vi "UI Main.vi"() -> ()   [LabVIEW 2013]
uses:
  controls/Control Configuration.ctl
  controls/UI Data.ctl
  controls/All FPGA Configuration Values.ctl
  controls/FPGA State.ctl
  controls/Raw Values.ctl
  Globals/Global - All UI Loop Stop.vi
  Globals/Global - UI Stream and Variable Connections.vi
  Globals/Global - Configuration Options.vi
  support/User Event - Stop/User Event - Stop.lvlib
  support/Message Queue/Message Queue.lvlib
panel:
  out "crio-9075-01.me.wisc.edu":string="128.104.188.88"
  in  "Switch to Safe State":bool
  in  "Exit":bool
  out "System Status":string
  out "Current FPGA Control Mode":u16(ring) items=["Safe State", "Manual", "Control (PID)"]
  in  "Settings Tab":T1(tab)
  in  "Channel 3 Setpoint":fxp<+/-,16,5>
  in  "Channel 2 Setpoint":fxp<+/-,16,5>
  in  "Channel 1 Setpoint":fxp<+/-,16,5>
  in  "Channel 0 Setpoint":fxp<+/-,16,5>
  in  "Update Control Configuration":bool
  in  "Control Configurations":T2[](array[typedef])
  in  "Run Control":bool
  in  "Stop Control":bool
  in  "Custom Controller Inputs":T3
  in  "Channel 3 Manual Value":fxp<+/-,16,5>
  in  "Channel 2 Manual Value":fxp<+/-,16,5>
  in  "Channel 1 Manual Value":fxp<+/-,16,5>
  in  "Channel 0 Manual Value":fxp<+/-,16,5>
  in  "Run Manual":bool
  in  "Stop Manual":bool
  out "Input Values":T4(graph)
  out "Output Values":T4(graph)
  out "Actual Loop Period (ticks)":u32
  out "Largest Contiguous Memory (bytes)":dbl(graph)
  out "CPU Usage (%)":dbl(graph)
  out "Connected?":bool
  in  "Connect to Controller":bool
  in  "Controller Address":string="128.104.188.88"
  # "LabVIEW FPGA Control on CompactRIO"
  # "Position Command"
  # "Connection Settings"
  # "Force Command"
  # "Element 0 - Chan 0\nElement 1 - Chan 1\nElement 2 - Chan 2\nElement 3 - Chan 3"
  # "Setpoint changes are sent to the target automatically."
  # "Control Configuration changes are sent to the target when you click \"Update Control Configurations\"."
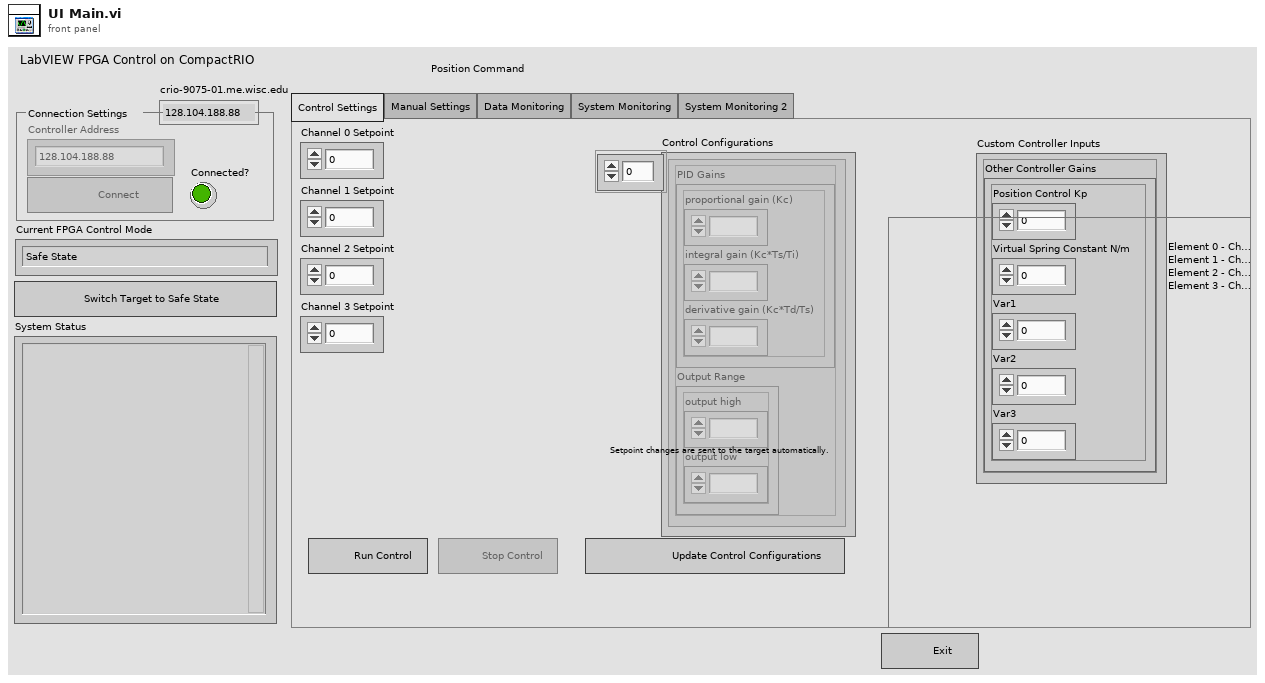
[diagram p1: front panel]
types:
  T1 = enum32{"Control Settings", "Manual Settings", "Data Monitoring", "System Monitoring", "System Monitoring 2"}
  T2 = typedef "Control Configuration.ctl" = cluster{"PID Gains":cluster{"proportional gain (Kc)":fxp<+/-,16,8>, "integral gain (Kc*Ts/Ti)":fxp<+/-,16,8>, "derivative gain (Kc*Td/Ts)":fxp<+/-,16,8>}, "Output Range":cluster{"output high":fxp<+/-,16,5>, "output low":fxp<+/-,16,5>}}
  T3 = cluster{"Other Controller Gains":cluster{"Position Control Kp":fxp<+/-,16,8>, "Virtual Spring Constant N/m":fxp<+/-,16,8>, "Var1":fxp<+/-,16,8>, "Var2":fxp<+/-,16,5>, "Var3":fxp<+/-,16,5>}}
  T4 = cluster{"Channel 0":dbl, "Channel 1":dbl, "Channel 2":dbl, "Channel 3":dbl}
  T5 = typedef "UI Data.ctl" = cluster{"Switch to Safe State Ref":refnum<vi>, "Run Manual Ref":refnum<vi>, "Stop Manual Ref":refnum<vi>, "Run Control Ref":refnum<vi>, "Stop Control Ref":refnum<vi>, "Update Control Configurations Ref":refnum<vi>, "Ch 0 Setpoint Ref":refnum<vi>, "Ch 1 Setpoint Ref":refnum<vi>, "Ch 2 Setpoint Ref":refnum<vi>, "Ch 3 Setpoint Ref":refnum<vi>, "Ch 0 Manual Ref":refnum<vi>, "Ch 1 Manual Ref":refnum<vi>, "Ch 2 Manual Ref":refnum<vi>, "Ch 3 Manual Ref":refnum<vi>, "Control Configurations Ref":refnum<vi>, "Custom Controller Cluster Ref":refnum<vi>}
  T6 = typedef "Message Queue.lvlib/All Message Queues.ctl" = cluster{"UI":refnum<queue>}
  T7 = cluster{"Channel 0 Setpoint":fxp<+/-,16,5>, "Channel 1 Setpoint":fxp<+/-,16,5>, "Channel 2 Setpoint":fxp<+/-,16,5>, "Channel 3 Setpoint":fxp<+/-,16,5>}
  T8 = cluster{"Channel 0 Manual Value":fxp<+/-,16,5>, "Channel 1 Manual Value":fxp<+/-,16,5>, "Channel 2 Manual Value":fxp<+/-,16,5>, "Channel 3 Manual Value":fxp<+/-,16,5>}
  T9 = cluster{"Message":string, "Message Data":variant}
  T10 = typedef "All FPGA Configuration Values.ctl" = cluster{"FPGA State":T11, "Manual Values":T12, "Setpoints":T12, "Control Configurations":T2[]}
  T11 = typedef "FPGA State.ctl" = enum16{"Safe State", "Manual", "Control (PID)"}
  T12 = typedef "Raw Values.ctl" = cluster{"Channel 0":fxp<+/-,20,5>, "Channel 1":fxp<+/-,20,5>, "Channel 2":fxp<+/-,20,5>, "Channel 3":fxp<+/-,20,5>}
  T13 = typedef "Variable References.ctl" = cluster{"CPU Usage":refnum<k21>, "Contiguous Memory":refnum<k21>, "Input Values":refnum<k21>, "Output Values":refnum<k21>, "FPGA Mode":refnum<k21>, "Actual Loop Period":refnum<k21>}
  T14 = cluster{string, "Custom Controller Inputs":cluster{"Other Controller Gains":cluster{"Position Control Kp":fxp<+/-,16,8>, "Virtual Spring Constant N/m":fxp<+/-,16,8>, "Var1":fxp<+/-,16,8>, "Var2":fxp<+/-,16,5>, "Var3":fxp<+/-,16,5>}}}
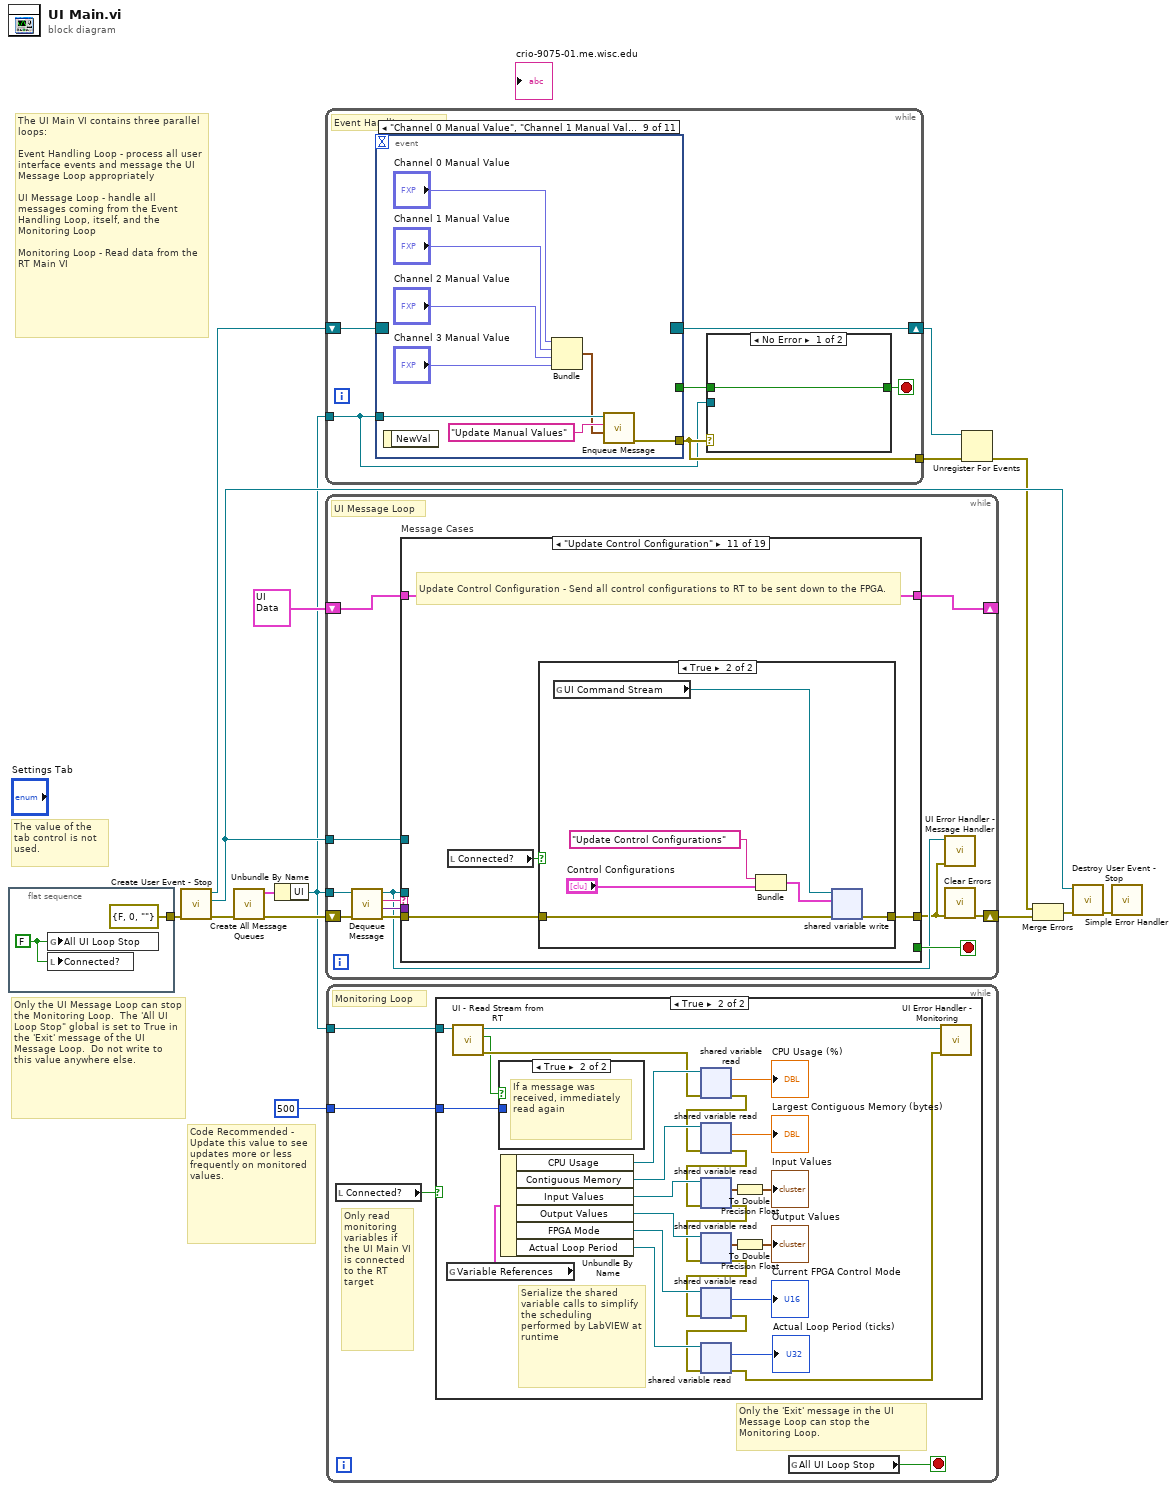
[diagram p0: block diagram]
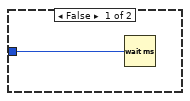
[diagram p2: hidden frame]
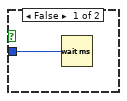
[diagram p3: hidden frame]
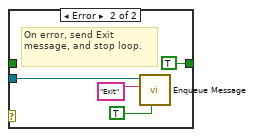
[diagram p4: hidden frame]
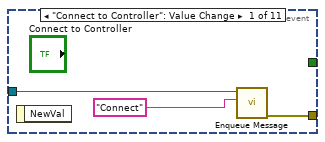
[diagram p5: hidden frame]
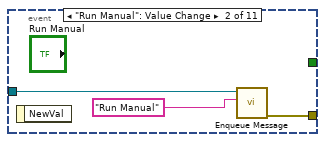
[diagram p6: hidden frame]
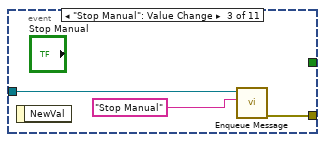
[diagram p7: hidden frame]
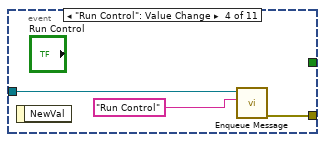
[diagram p8: hidden frame]
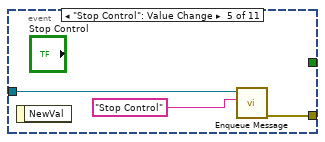
[diagram p9: hidden frame]
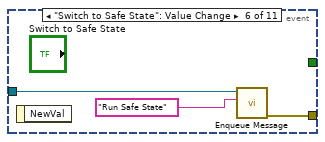
[diagram p10: hidden frame]
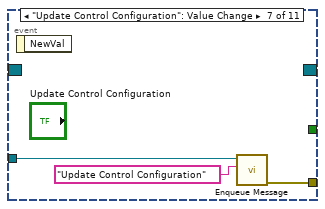
[diagram p11: hidden frame]
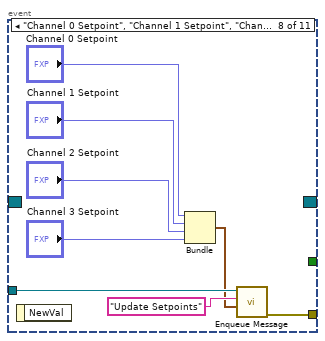
[diagram p12: hidden frame]
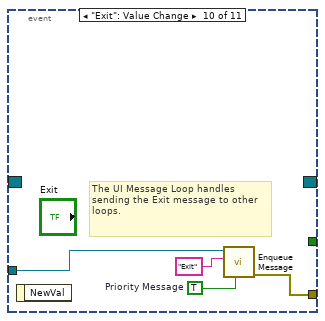
[diagram p13: hidden frame]
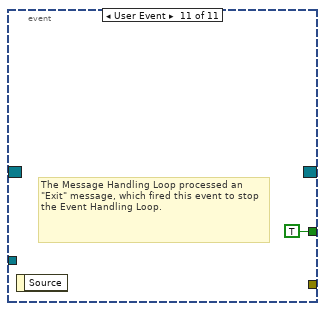
[diagram p14: hidden frame]
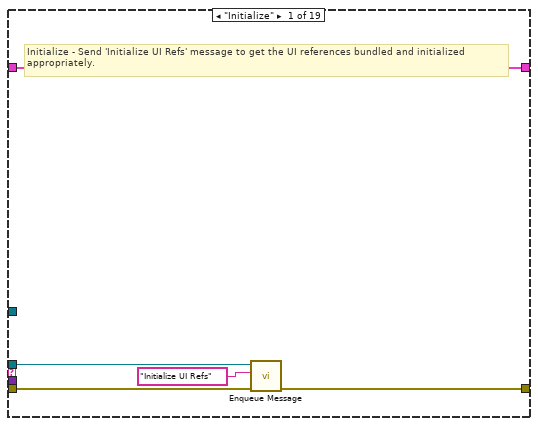
[diagram p15: hidden frame]
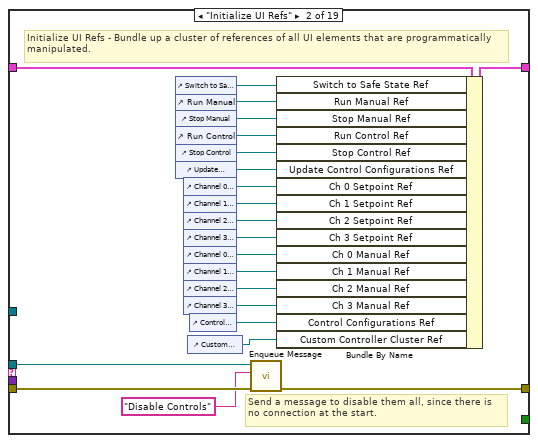
[diagram p16: hidden frame]
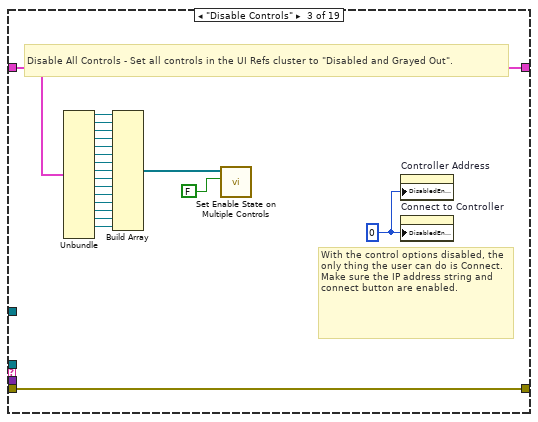
[diagram p17: hidden frame]
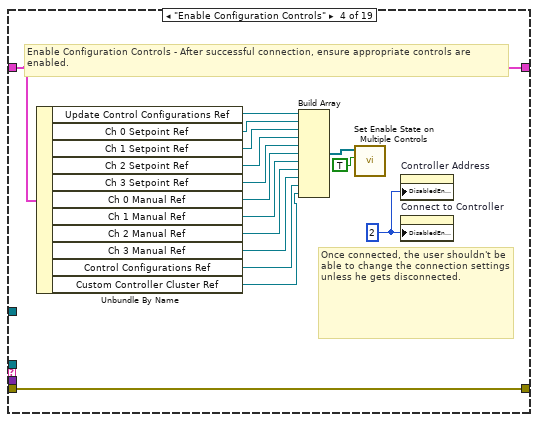
[diagram p18: hidden frame]
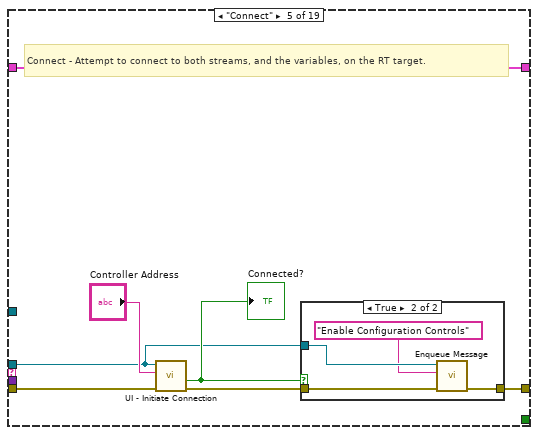
[diagram p19: hidden frame]
diagram:
  # "Code Recommended - Update this value to see updates more or less frequently on monitored values."
  # "The UI Main VI contains three parallel loops:\n\nEvent Handling Loop - process all user interface events and message the UI Message Loop appropriately\n\nUI Message Loop - handle all messages coming from the Event Handling Loop, itself, and the Monitoring Loop\n\nMonitoring Loop - Read data from the RT Main VI"
  # "The value of the tab control is not used."
  # "Only the UI Message Loop can stop the Monitoring Loop.  The 'All UI Loop Stop\" global is set to True in the 'Exit' message of the UI Message Loop.  Do not write to this value anywhere else."
  n1 = flat-sequence {
    tunnel: [errorcluster {"status"=FALSE, "code"=0, "source"=""} ("error in (no error)")] -> w2
    frame #0 {
      w16 = FALSE
      n2 = global write "Global - All UI Loop Stop.vi" "All UI Loop Stop"(w16) -> ()
      n3 = local write "Connected?"(w16) -> ()
    }
  }
  n4 = call "Create User Event - Stop.vi"("error in (no error)"=w2) -> ("error out"=w10:errorcluster, "User Event - Stop"=w11:refnum<user-event>, "Stop Event Registration Refnum"=w12:refnum<event-registration>)  [unwired: 8 in]
  n5 = call "Create All Message Queues.vi"("error in (no error)"=w10) -> ("error out"=w8:errorcluster, "Message Queues out"=w9:T6)  [unwired: 9 in]
  n6 = Unbundle By Name(w9) -> ("UI"=w3:refnum<queue>)
  n7 = while {
    tunnel: w3 -> [w19]
    tunnel: [w21] -> w14
    shift-right: [w18] -> w6
    shift-left: w12 -> [w20]
    stop <- w22 stop-if-true
    # "Event Handling Loop"
    n8 = event shown="[8] \"Channel 0 Manual Value\", \"Channel 1 Manual Value\", \"Channel 2 Manual Value\", \"Channel 3 Manual Value\": Value Change" {
      selector: w20 -> [_ _ _ _ _ _ _ _ _ _ _]
      dyn-events: [_ _ _ _ _ _ _ _ _ _ _] -> w18
      timeout: _ -> [_ _ _ _ _ _ _ _ _ _ _]
      tunnel: [_ _ _ _ _ _ _ _ _ _ TRUE ("Discard?")] -> w23
      tunnel: w19 -> [w29 w32 w35 w38 w41 w44 w49 w52 w61 w66 _]
      tunnel: [w31 w34 w37 w40 w43 w46 w48 w51 w60 w69 _] -> w21
      event "Connect to Controller": Value Change {
        n9 = event-data() -> ()  [unwired: 1 in, 1 out]
        n10 = call "Enqueue Message.vi"("Message"="Connect", "Message Queue"=w29) -> ("error out"=w31:errorcluster)  [unwired: 8 in, 1 out]
      }
      event "Run Manual": Value Change {
        n11 = event-data() -> ()  [unwired: 1 in, 1 out]
        n12 = call "Enqueue Message.vi"("Message"="Run Manual", "Message Queue"=w32) -> ("error out"=w34:errorcluster)  [unwired: 8 in, 1 out]
      }
      event "Stop Manual": Value Change {
        n13 = event-data() -> ()  [unwired: 1 in, 1 out]
        n14 = call "Enqueue Message.vi"("Message"="Stop Manual", "Message Queue"=w35) -> ("error out"=w37:errorcluster)  [unwired: 8 in, 1 out]
      }
      event "Run Control": Value Change {
        n15 = event-data() -> ()  [unwired: 1 in, 1 out]
        n16 = call "Enqueue Message.vi"("Message"="Run Control", "Message Queue"=w38) -> ("error out"=w40:errorcluster)  [unwired: 8 in, 1 out]
      }
      event "Stop Control": Value Change {
        n17 = event-data() -> ()  [unwired: 1 in, 1 out]
        n18 = call "Enqueue Message.vi"("Message"="Stop Control", "Message Queue"=w41) -> ("error out"=w43:errorcluster)  [unwired: 8 in, 1 out]
      }
      event "Switch to Safe State": Value Change {
        n19 = event-data() -> ()  [unwired: 1 in, 1 out]
        n20 = call "Enqueue Message.vi"("Message"="Run Safe State", "Message Queue"=w44) -> ("error out"=w46:errorcluster)  [unwired: 8 in, 1 out]
      }
      event "Update Control Configuration": Value Change {
        n21 = event-data() -> ()  [unwired: 1 in, 1 out]
        n22 = call "Enqueue Message.vi"("Message"="Update Control Configuration", "Message Queue"=w49) -> ("error out"=w48:errorcluster)  [unwired: 8 in, 1 out]
      }
      event "Channel 0 Setpoint", "Channel 1 Setpoint", "Channel 2 Setpoint", "Channel 3 Setpoint": Value Change {
        n23 = event-data() -> ()  [unwired: 1 in, 1 out]
        n24 = Bundle("Channel 0 Setpoint"="Channel 0 Setpoint", "Channel 1 Setpoint"="Channel 1 Setpoint", "Channel 2 Setpoint"="Channel 2 Setpoint", "Channel 3 Setpoint"="Channel 3 Setpoint") -> (w50:T7)  [unwired: 1 in]
        n25 = call "Enqueue Message.vi"("Message Data"=w50, "Message"="Update Setpoints", "Message Queue"=w52) -> ("error out"=w51:errorcluster)  [unwired: 7 in, 1 out]
      }
      event "Channel 0 Manual Value", "Channel 1 Manual Value", "Channel 2 Manual Value", "Channel 3 Manual Value": Value Change {
        n26 = event-data() -> ()  [unwired: 1 in, 1 out]
        n27 = Bundle("Channel 0 Manual Value"="Channel 0 Manual Value", "Channel 1 Manual Value"="Channel 1 Manual Value", "Channel 2 Manual Value"="Channel 2 Manual Value", "Channel 3 Manual Value"="Channel 3 Manual Value") -> (w58:T8)  [unwired: 1 in]
        n28 = call "Enqueue Message.vi"("Message Data"=w58, "Message"="Update Manual Values", "Message Queue"=w61) -> ("error out"=w60:errorcluster)  [unwired: 7 in, 1 out]
      }
      event "Exit": Value Change {
        w67 = TRUE  # Priority Message
        # "The UI Message Loop handles sending the Exit message to other loops."
        n29 = event-data() -> ()  [unwired: 1 in, 1 out]
        n30 = call "Enqueue Message.vi"("Priority Message? (F)"=w67, "Message"="Exit", "Message Queue"=w66) -> ("error out"=w69:errorcluster)  [unwired: 7 in, 1 out]
      }
      event User Event {
        # "The Message Handling Loop processed an \"Exit\" message, which fired this event to stop the Event Handling Loop."
        n31 = event-data() -> ()  [unwired: 1 in, 1 out]
      }
    }
    n32 = case shown="No Error" w21 {
      tunnel: [w24 TRUE ("Discard?")] -> w22
      tunnel: w23 -> [w24 _]
      tunnel: w19 -> [_ w25]
      frame No Error {
      }
      frame Error {
        # "On error, send Exit message, and stop loop."
        n33 = call "Enqueue Message.vi"("Priority Message? (F)"=TRUE ("Discard?"), "Message"="Exit", "Message Queue"=w25) -> ()  [unwired: 7 in, 2 out]
      }
    }
  }
  n34 = while {
    tunnel: w3 -> [w76]
    tunnel: w11 -> [w81]
    shift-right: [w71] -> w15
    shift-left: w8 -> [w80]
    shift-right: [w74] -> _
    shift-left: T5 {"Switch to Safe State Ref"=refnum, "Run Manual Ref"=refnum, "Stop Manual Ref"=refnum, "Run Control Ref"=refnum, "Stop Control Ref"=refnum, "Update Control Configurations Ref"=refnum, "Ch 0 Setpoint Ref"=refnum, "Ch 1 Setpoint Ref"=refnum, "Ch 2 Setpoint Ref"=refnum, "Ch 3 Setpoint Ref"=refnum, "Ch 0 Manual Ref"=refnum, "Ch 1 Manual Ref"=refnum, "Ch 2 Manual Ref"=refnum, "Ch 3 Manual Ref"=refnum, "Control Configurations Ref"=refnum, "Custom Controller Cluster Ref"=refnum} ("Measurement UI Controls") -> [w75]
    stop <- w82 stop-if-true
    # "UI Message Loop"
    n35 = call "Dequeue Message.vi"("error in (no error)"=w80, "Message Queue"=w76) -> ("error out"=w79:errorcluster, "Message Data"=w77:variant, "Message"=w78:string, "dup Message Queue"=w73:refnum<queue>)  [unwired: 6 in]
    n36 = case "Message Cases" shown="\"Update Control Configuration\"" w78 {
      selector: w78 -> [_ _ _ _ _ _ _ _ _ w207 _ _ w250 _ w300 _ _ _ w361]
      tunnel: w73 -> [w84 w91 _ _ w147 _ w165 _ w179 w208 _ _ _ _ w304 _ w346 _ _]
      tunnel: w79 -> [w86 w109 w129 w131 w152 w163 w167 w172 w203 w210 w228 w239 w251 w271 w314 w335 w351 w356 _]
      tunnel: [w85 w92 w129 w131 w146 w163 w166 w171 w182 w209 w227 w238 w252 w270 w315 w333 w352 w355 w359] -> w72
      tunnel: [_ _ _ _ _ _ _ _ _ _ _ _ _ _ _ _ TRUE _ _] -> w82
      tunnel: w77 -> [_ _ _ _ _ _ _ _ w201 _ _ _ w249 w269 w312 w332 _ _ _]
      tunnel: w81 -> [_ _ _ _ _ _ _ _ _ _ _ _ _ _ _ _ w350 _ _]
      tunnel: w75 -> [w87 w108 w128 w142 w151 w162 w169 w173 w198 w211 w229 w240 w253 w268 w316 w334 w348 w354 w357]
      tunnel: [w87 w107 w128 w142 w151 w162 w169 w173 w198 w211 w229 w240 w253 w268 w316 w334 w348 w354 w357] -> w74
      frame "Initialize" {
        # "Initialize - Send 'Initialize UI Refs' message to get the UI references bundled and initialized appropriately."
        n37 = call "Enqueue Message.vi"("error in (no error)"=w86, "Message"="Initialize UI Refs", "Message Queue"=w84) -> ("error out"=w85:errorcluster)  [unwired: 7 in, 1 out]
      }
      frame "Initialize UI Refs" {
        # "Send a message to disable them all, since there is no connection at the start."
        # "Initialize UI Refs - Bundle up a cluster of references of all UI elements that are programmatically manipulated."
        n38 = control-ref of="Switch to Safe State"() -> (w106:refnum<vi>)
        n39 = control-ref of="Run Manual"() -> (w105:refnum<vi>)
        n40 = control-ref of="Stop Manual"() -> (w104:refnum<vi>)
        n41 = control-ref of="Run Control"() -> (w103:refnum<vi>)
        n42 = control-ref of="Stop Control"() -> (w102:refnum<vi>)
        n43 = control-ref of="Update Control Configuration"() -> (w101:refnum<vi>)
        n44 = control-ref of="Channel 0 Setpoint"() -> (w100:refnum<vi>)
        n45 = control-ref of="Channel 1 Setpoint"() -> (w99:refnum<vi>)
        n46 = control-ref of="Channel 2 Setpoint"() -> (w98:refnum<vi>)
        n47 = control-ref of="Channel 3 Setpoint"() -> (w97:refnum<vi>)
        n48 = control-ref of="Channel 0 Manual Value"() -> (w96:refnum<vi>)
        n49 = control-ref of="Channel 1 Manual Value"() -> (w95:refnum<vi>)
        n50 = control-ref of="Channel 2 Manual Value"() -> (w94:refnum<vi>)
        n51 = control-ref of="Channel 3 Manual Value"() -> (w93:refnum<vi>)
        n52 = control-ref of="Custom Controller Inputs"() -> (w88:refnum<vi>)
        n53 = control-ref of="Control Configurations"() -> (w89:refnum<vi>)
        n54 = call "Enqueue Message.vi"("error in (no error)"=w109, "Message"="Disable Controls", "Message Queue"=w91) -> ("error out"=w92:errorcluster)  [unwired: 7 in, 1 out]
        n55 = Bundle By Name(cluster=w108, "Switch to Safe State Ref"=w106, "Run Manual Ref"=w105, "Stop Manual Ref"=w104, "Run Control Ref"=w103, "Stop Control Ref"=w102, "Update Control Configurations Ref"=w101, "Ch 0 Setpoint Ref"=w100, "Ch 1 Setpoint Ref"=w99, "Ch 2 Setpoint Ref"=w98, "Ch 3 Setpoint Ref"=w97, "Ch 0 Manual Ref"=w96, "Ch 1 Manual Ref"=w95, "Ch 2 Manual Ref"=w94, "Ch 3 Manual Ref"=w93, "Control Configurations Ref"=w89, "Custom Controller Cluster Ref"=w88) -> (w107:T5)
      }
      frame "Disable Controls" {
        w110 = 0
        # "With the control options disabled, the only thing the user can do is Connect. Make sure the IP address string and connect button are enabled."
        # "Disable All Controls - Set all controls in the UI Refs cluster to \"Disabled and Grayed Out\"."
        n56 = Unbundle(w128) -> ("Switch to Safe State Ref"=w127:refnum<vi>, "Run Manual Ref"=w126:refnum<vi>, "Stop Manual Ref"=w125:refnum<vi>, "Run Control Ref"=w124:refnum<vi>, "Stop Control Ref"=w123:refnum<vi>, "Update Control Configurations Ref"=w122:refnum<vi>, "Ch 0 Setpoint Ref"=w121:refnum<vi>, "Ch 1 Setpoint Ref"=w120:refnum<vi>, "Ch 2 Setpoint Ref"=w119:refnum<vi>, "Ch 3 Setpoint Ref"=w118:refnum<vi>, "Ch 0 Manual Ref"=w117:refnum<vi>, "Ch 1 Manual Ref"=w116:refnum<vi>, "Ch 2 Manual Ref"=w115:refnum<vi>, "Ch 3 Manual Ref"=w114:refnum<vi>, "Control Configurations Ref"=w113:refnum<vi>)  [unwired: 1 out]
        n57 = Build Array(w127, w126, w125, w124, w123, w122, w121, w120, w119, w118, w117, w116, w115, w114, w113) -> (w112:refnum<vi>[])
        n58 = call "Set Enable State on Multiple Controls.vi"("Enable?"=FALSE, "Controls"=w112) -> ()  [unwired: 10 in]
        n59 = property on="Controller Address" class="Str"("DisabledEnum"=w110) -> ()  [unwired: 2 in, 2 out]
        n60 = property on="Connect to Controller" class="Bool"("DisabledEnum"=w110) -> ()  [unwired: 2 in, 2 out]
      }
      frame "Enable Configuration Controls" {
        w143 = 2
        # "Once connected, the user shouldn't be able to change the connection settings unless he gets disconnected."
        # "Enable Configuration Controls - After successful connection, ensure appropriate controls are enabled."
        n61 = Unbundle By Name(w142) -> ("Update Control Configurations Ref"=w141:refnum<vi>, "Ch 0 Setpoint Ref"=w140:refnum<vi>, "Ch 1 Setpoint Ref"=w139:refnum<vi>, "Ch 2 Setpoint Ref"=w138:refnum<vi>, "Ch 3 Setpoint Ref"=w137:refnum<vi>, "Ch 0 Manual Ref"=w136:refnum<vi>, "Ch 1 Manual Ref"=w135:refnum<vi>, "Ch 2 Manual Ref"=w134:refnum<vi>, "Ch 3 Manual Ref"=w133:refnum<vi>, "Control Configurations Ref"=w132:refnum<vi>, "Custom Controller Cluster Ref"=w130:refnum<vi>)
        n62 = Build Array(w141, w140, w139, w138, w137, w136, w135, w134, w133, w132, w130) -> (w145:refnum<vi>[])
        n63 = call "Set Enable State on Multiple Controls.vi"("Enable?"=TRUE, "Controls"=w145) -> ()  [unwired: 10 in]
        n64 = property on="Controller Address" class="Str"("DisabledEnum"=w143) -> ()  [unwired: 2 in, 2 out]
        n65 = property on="Connect to Controller" class="Bool"("DisabledEnum"=w143) -> ()  [unwired: 2 in, 2 out]
      }
      frame "Connect" {
        # "Connect - Attempt to connect to both streams, and the variables, on the RT target."
        n66 = call "UI - Initiate Connection.vi"("error in (no error)"=w152, "Controller Address"="Controller Address", "Message Queue"=w147) -> ("error out"=w149:errorcluster, "Connected?"=w148:bool)  [unwired: 7 in]
        "Connected?" <- w148
        n67 = case shown="True" w148 {
          tunnel: w149 -> [w153 w157]
          tunnel: w147 -> [_ w156]
          tunnel: [w153 w155] -> w146
          frame False {
          }
          frame True {
            n68 = call "Enqueue Message.vi"("error in (no error)"=w157, "Message"="Enable Configuration Controls", "Message Queue"=w156) -> ("error out"=w155:errorcluster)  [unwired: 7 in, 1 out]
          }
        }
      }
      frame "Close Connections" {
        # "Close Connections - Close the connections shared with the Monitoring Loop."
        n69 = global read "Global - UI Stream and Variable Connections.vi" "UI Command Stream"() -> (w161:refnum<k21>)
        n70 = global read "Global - UI Stream and Variable Connections.vi" "RT Message Stream"() -> (w160:refnum<k21>)
        n71 = global read "Global - UI Stream and Variable Connections.vi" "Variable References"() -> (w159:T13)
        n72 = local write "Connected?"(FALSE ("Connected?")) -> ()
        n73 = Destroy Stream Endpoint(11:w161) -> ()  [unwired: 1 in, 1 out]
        n74 = Destroy Stream Endpoint(11:w160) -> ()  [unwired: 1 in, 1 out]
        n75 = call "Close Variable Connections.vi"("Variable References"=w159) -> ()  [unwired: 11 in]
      }
      frame "Disconnect UI" {
        # "Disconnect UI - Something has gone wrong with the connection. Reinitialize the UI to its disconnected state."
        n76 = local write "Connected?"(FALSE ("Connected?")) -> ()
        n77 = call "Enqueue Message.vi"("error in (no error)"=w167, "Message"="Disable Controls", "Message Queue"=w165) -> ("error out"=w166:errorcluster)  [unwired: 7 in, 1 out]
      }
      frame "Get Settings from FPGA" {
        # "Get Settings from FPGA - Send a command to the RT to retrieve all current FPGA Main VI parameter values and send them back to the UI."
        n78 = local read "Connected?"() -> (w170:bool)
        n79 = case shown="True" w170 {
          tunnel: w172 -> [w174 w178]
          tunnel: [w174 w177] -> w171
          frame False {
            # "Don't bother trying to send a message to the RT system if UI Main VI isn't even connected"
          }
          frame True {
            n80 = global read "Global - UI Stream and Variable Connections.vi" "UI Command Stream"() -> (w175:refnum<k21>)
            n81 = shared-variable-write(w175, w178, T9 {"Message"="Send FPGA Configuration to UI", "Message Data"=variant} ("data in")) -> (w177:errorcluster)  [unwired: 1 in, 2 out]
          }
        }
      }
      frame "Initial UI Values" {
        # "Initial UI Values - These are the current values of the FPGA Main VI's R/W controls. They are used to initialize the panel of UI Main VI upon successful connection to the RT target."
        # "Set values of all manual and setpoint controls via reference."
        n82 = Variant To Data(error in=w203, type=T10 {"FPGA State"=enum."Safe State", "Manual Values"={"Channel 0"=0.0, "Channel 1"=0.0, "Channel 2"=0.0, "Channel 3"=0.0}, "Setpoints"={"Channel 0"=0.0, "Channel 1"=0.0, "Channel 2"=0.0, "Channel 3"=0.0}, "Control Configurations"=[]} ("All FPGA Configuration Values"), Variant=w201) -> (data=w199:T10, error out=w202:errorcluster)
        n83 = Unbundle By Name(w198) -> ("Ch 0 Setpoint Ref"=w193:refnum<vi>, "Ch 1 Setpoint Ref"=w192:refnum<vi>, "Ch 2 Setpoint Ref"=w191:refnum<vi>, "Ch 3 Setpoint Ref"=w190:refnum<vi>, "Ch 0 Manual Ref"=w189:refnum<vi>, "Ch 1 Manual Ref"=w188:refnum<vi>, "Ch 2 Manual Ref"=w187:refnum<vi>, "Ch 3 Manual Ref"=w186:refnum<vi>)
        n84 = Unbundle By Name(w199) -> ("Setpoints"=w197:T12, "Manual Values"=w196:T12, "Control Configurations"=w183:T2[], "FPGA State"=w180:T11)
        n85 = Build Array(w193, w192, w191, w190, w189, w188, w187, w186) -> (w185:refnum<vi>[])
        n86 = Cluster To Array(cluster=w197) -> (array=w195:fxp<+/-,20,5>[])
        n87 = Cluster To Array(cluster=w196) -> (array=w194:fxp<+/-,20,5>[])
        n88 = local write "Current FPGA Control Mode"(w180) -> ()
        n89 = Build Array (concatenate)(w195, w194) -> (w184:fxp<+/-,20,5>[])
        n90 = local write "Control Configurations"(w183) -> ()
        n91 = for {
          tunnel: w185 -> [w205] mode=indexing
          tunnel: w184 -> [w204] mode=indexing
          n92 = property class="DigNum"(reference=w205, "Value"=w204) -> ()  [unwired: 1 in, 2 out]
        }
        n93 = call "Enqueue Message.vi"("error in (no error)"=w202, "Message Data"=w180, "Message"="Update Display Mode", "Message Queue"=w179) -> ("error out"=w182:errorcluster)  [unwired: 6 in, 1 out]
      }
      frame "Run Control", "Run Manual", "Run Safe State", "Stop Control", "Stop Manual" {
        # "Run/Stop buttons - Send a command to switch the FPGA into the appropriate state. Send a message to update this UI to reflect the new state."
        n94 = local read "Connected?"() -> (w206:bool)
        n95 = case shown="True" w206 {
          tunnel: w210 -> [w212 w222]
          tunnel: [w212 w218] -> w209
          tunnel: w208 -> [_ w217]
          tunnel: w207 -> [_ w216]
          frame False {
            # "Don't bother trying to send a message to the RT system if UI Main VI isn't even connected"
          }
          frame True {
            # "Run Manual and Run Control switch into their respective states. Anything else switches to Safe State."
            n96 = case shown="\"Safe State\", \"Stop Control\", \"Stop Manual\", Default" w216 {
              tunnel: [FPGA_State."Safe State" ("FPGA State") FPGA_State."Control (PID)" ("FPGA State") FPGA_State."Manual" ("FPGA State")] -> w213
              frame "Safe State", "Stop Control", "Stop Manual", Default {
              }
              frame "Run Control" {
              }
              frame "Run Manual" {
              }
            }
            n97 = global read "Global - UI Stream and Variable Connections.vi" "UI Command Stream"() -> (w214:refnum<k21>)
            n98 = Bundle("Update FPGA State", "FPGA State"=w213) -> (w219:cluster{string, "FPGA State":T11})  [unwired: 1 in]
            n99 = shared-variable-write(w214, w222, w219) -> (w221:errorcluster)  [unwired: 1 in, 2 out]
            n100 = call "Enqueue Message.vi"("error in (no error)"=w221, "Message Data"=w213, "Message"="Update Display Mode", "Message Queue"=w217) -> ("error out"=w218:errorcluster)  [unwired: 6 in, 1 out]
          }
        }
      }
      frame "Update Control Configuration" {
        # "Update Control Configuration - Send all control configurations to RT to be sent down to the FPGA."
        n101 = local read "Connected?"() -> (w226:bool)
        n102 = case shown="True" w226 {
          tunnel: w228 -> [w230 w236]
          tunnel: [w230 w235] -> w227
          frame False {
            # "Don't bother trying to send a message to the RT system if UI Main VI isn't even connected"
          }
          frame True {
            n103 = global read "Global - UI Stream and Variable Connections.vi" "UI Command Stream"() -> (w231:refnum<k21>)
            n104 = Bundle("Update Control Configurations", "Control Configurations"="Control Configurations") -> (w233:cluster{string, "Control Configurations":T2[]})  [unwired: 1 in]
            n105 = shared-variable-write(w231, w236, w233) -> (w235:errorcluster)  [unwired: 1 in, 2 out]
          }
        }
      }
      frame "Update Custom Controller" {
        # "Update Control Configuration - Send all control configurations to RT to be sent down to the FPGA."
        n106 = local read "Connected?"() -> (w237:bool)
        n107 = case shown="True" w237 {
          tunnel: w239 -> [w241 w247]
          tunnel: [w241 w246] -> w238
          frame False {
            # "Don't bother trying to send a message to the RT system if UI Main VI isn't even connected"
          }
          frame True {
            n108 = global read "Global - UI Stream and Variable Connections.vi" "UI Command Stream"() -> (w243:refnum<k21>)
            n109 = Bundle("\"Update Custom Controller\"", "Custom Controller Inputs"="Custom Controller Inputs") -> (w244:T14)  [unwired: 1 in]
            n110 = shared-variable-write(w243, w247, w244) -> (w246:errorcluster)  [unwired: 1 in, 2 out]
          }
        }
      }
      frame "Update Manual Values", "Update Setpoints" {
        # "Update Manual Values/Setpoints - Send all manual values/setpoints to RT to be sent down to the FPGA."
        n111 = local read "Connected?"() -> (w248:bool)
        n112 = case shown="True" w248 {
          tunnel: [w254 w260] -> w252
          tunnel: w251 -> [w254 w258]
          tunnel: w250 -> [_ w257]
          tunnel: w249 -> [_ w256]
          frame False {
            # "Don't bother trying to send a message to the RT system if UI Main VI isn't even connected"
          }
          frame True {
            n113 = global read "Global - UI Stream and Variable Connections.vi" "UI Command Stream"() -> (w255:refnum<k21>)
            n114 = Bundle(w257, "Message Data"=w256) -> (w259:cluster{string, "Message Data":variant})  [unwired: 1 in]
            n115 = shared-variable-write(w255, w258, w259) -> (w260:errorcluster)  [unwired: 1 in, 2 out]
          }
        }
      }
      frame "Update Display Mode" {
        # "Update Display Mode - Enable/Disable Controls appropriately for the new display mode."
        n116 = Variant To Data(error in=w271, type=FPGA_State."Safe State" ("FPGA State"), Variant=w269) -> (data=w267:T11, error out=w270:errorcluster)
        n117 = Unbundle By Name(w268) -> ("Switch to Safe State Ref"=w266:refnum<vi>, "Run Manual Ref"=w265:refnum<vi>, "Stop Manual Ref"=w264:refnum<vi>, "Run Control Ref"=w263:refnum<vi>, "Stop Control Ref"=w262:refnum<vi>)
        n118 = case shown="\"Control (PID)\"" w267 {
          tunnel: w266 -> [w276 w285 w292]
          tunnel: w265 -> [w272 w284 w294]
          tunnel: w264 -> [w275 w283 w291]
          tunnel: w263 -> [w274 w281 w293]
          tunnel: w262 -> [w273 w282 w290]
          frame "Control (PID)" {
            n119 = Build Array "Controls to Enable"(w276, w273, w272) -> (w280:refnum<vi>[])
            n120 = Build Array "Controls to Disable"(w275, w274) -> (w278:refnum<vi>[])
            n121 = call "Set Enable State on Multiple Controls.vi"("Enable?"=FALSE, "Controls"=w278) -> ()  [unwired: 10 in]
            n122 = call "Set Enable State on Multiple Controls.vi"("Enable?"=TRUE, "Controls"=w280) -> ()  [unwired: 10 in]
          }
          frame "Manual" {
            n123 = Build Array "Controls to Enable"(w285, w283, w281) -> (w289:refnum<vi>[])
            n124 = Build Array "Controls to Disable"(w284, w282) -> (w287:refnum<vi>[])
            n125 = call "Set Enable State on Multiple Controls.vi"("Enable?"=FALSE, "Controls"=w287) -> ()  [unwired: 10 in]
            n126 = call "Set Enable State on Multiple Controls.vi"("Enable?"=TRUE, "Controls"=w289) -> ()  [unwired: 10 in]
          }
          frame "Safe State" {
            # "This frame runs when FPGA is in Safe State. Only enable the two run buttons."
            n127 = Build Array "Controls to Enable"(w294, w293) -> (w298:refnum<vi>[])
            n128 = Build Array "Controls to Disable"(w292, w291, w290) -> (w296:refnum<vi>[])
            n129 = call "Set Enable State on Multiple Controls.vi"("Enable?"=FALSE, "Controls"=w296) -> ()  [unwired: 10 in]
            n130 = call "Set Enable State on Multiple Controls.vi"("Enable?"=TRUE, "Controls"=w298) -> ()  [unwired: 10 in]
          }
        }
      }
      frame "Critical Error", "Log-Only Error", "Non-Critical Error", "RT Error" {
        # "Error - Display message in status indicator on panel.  If it's a critical error, shut down this VI with an 'Exit' message."
        n131 = case shown="Default" w300 {
          selector: w300 -> [_ w318]
          tunnel: ["UI Error" w318] -> w299
          frame Default {
          }
          frame "RT Error" {
          }
        }
        n132 = Variant To Data(error in=w314, type=errorcluster {"status"=FALSE, "code"=0, "source"=""} ("error constant"), Variant=w312) -> (data=w307:errorcluster, error out=w313:errorcluster)
        n133 = Unbundle By Name(w307) -> ("code"=w306:i32, "source"=w310:string)
        n134 = Format Date/Time String() -> (date/time string=w309:string)  [unwired: 3 in]
        n135 = Format Into String(format string="\n%s: %s %d - %s", w309, w299, w306, w310) -> (resulting string=w301:string)  [unwired: 2 in, 1 out]
        n136 = call "Enqueue Message.vi"("error in (no error)"=w313, "Message Data"=w301, "Message"="Update System Status", "Message Queue"=w304) -> ("error out"=w305:errorcluster, "dup Message Queue"=w303:refnum<queue>)  [unwired: 6 in]
        n137 = case shown="Default" w300 {
          tunnel: w305 -> [w319 w323]
          tunnel: w303 -> [_ w321]
          tunnel: [w319 w322] -> w315
          frame Default {
          }
          frame "Critical Error" {
            n138 = call "Enqueue Message.vi"("error in (no error)"=w323, "Message"="Exit", "Message Queue"=w321) -> ("error out"=w322:errorcluster)  [unwired: 7 in, 1 out]
          }
        }
      }
      frame "Update System Status" {
        # "Code Recommended - The code below ensures that the System Status string value does not become too large.  It uses the same maximum size as the RT error log to determine whether or not to remove the last half of the log string. Change this logic if you wish to maintain more/less of the information in the System Status string."
        # "Update System Status - Add a new string to the beginning of the System Status string on the UI."
        n139 = Variant To Data(error in=w335, type="", Variant=w332) -> (data=w329:string, error out=w333:errorcluster)
        n140 = local read "System Status"() -> (w327:string)
        n141 = global read "Global - Configuration Options.vi" "Error Log Max Size (bytes)"() -> (w325:i64)
        n142 = String Length(string=w327) -> (length=w328:i32)
        n143 = Greater?(x=w328, y=w325) -> (0:w326:bool)
        n144 = case shown="True" w326 {
          tunnel: w327 -> [w336 w340]
          tunnel: w325 -> [_ w339]
          tunnel: [w336 w341] -> w324
          frame False {
          }
          frame True {
            n145 = Divide(x=w339, y=i64 2) -> (x/y=w338:dbl)
            n146 = String Subset(string=w340, length (rest)=w338) -> (substring=w341:string)  [unwired: 1 in]
          }
        }
        n147 = Concatenate Strings(w329, w324) -> (→"System Status":string)
      }
      frame "Exit" {
        # "Close all connections"
        # "Stop Monitoring Loop"
        # "Stop Event Handling Loop"
        # "Release the UI Message queue reference"
        # "Stop UI Message Loop"
        # "Exit - Fire the User Event to stop the Event Handling Loop, and toggle the local variable to stop the Monitoring Loop.  This message alone causes all three loops to stop."
        n148 = global write "Global - All UI Loop Stop.vi" "All UI Loop Stop"(TRUE ("Stop Monitoring Loop")) -> ()
        n149 = call "Fire User Event - Stop.vi"("User Event - Stop"=w350) -> ("error out"=w349:errorcluster)  [unwired: 10 in]
        n150 = Release Queue(queue=w346, error in (no error)=w351) -> (error out=w347:errorcluster)  [unwired: 1 in, 2 out]
        n151 = global read "Global - UI Stream and Variable Connections.vi" "UI Command Stream"() -> (w344:refnum<k21>)
        n152 = global read "Global - UI Stream and Variable Connections.vi" "RT Message Stream"() -> (w343:refnum<k21>)
        n153 = global read "Global - UI Stream and Variable Connections.vi" "Variable References"() -> (w342:T13)
        n154 = Destroy Stream Endpoint(11:w344) -> ()  [unwired: 1 in, 1 out]
        n155 = Destroy Stream Endpoint(11:w343) -> ()  [unwired: 1 in, 1 out]
        n156 = call "Close Variable Connections.vi"("Variable References"=w342) -> ()  [unwired: 11 in]
        n157 = Merge Errors(w349, w347) -> (w352:errorcluster)
      }
      frame "---Copy This Frame---" {
        # "Duplicate this frame when creating new messages.  Change this comment in the duplicated frame to describe this message."
        n158 = Merge Errors(w356) -> (w355:errorcluster)
      }
      frame Default {
        # "'Default' case only runs if there is a message that isn't defined in any of the other cases.  Output a programming error."
        n159 = Format Into String(format string="The invalid message string \"%s\" was received in the Message Handling Loop." ("Invalid Message Loop Message"), w361) -> (resulting string=w358:string)  [unwired: 2 in, 1 out]
        n160 = call <vilib>:"Error Cluster From Error Code.vi"("error message (\"\")"=w358, "error code (0)"=1) -> ("error out"=w359:errorcluster)  [unwired: 7 in]
      }
    }
    n161 = call "UI Error Handler - Message Handler.vi"("error in (no error)"=w72, "Message Queue"=w73) -> ()  [unwired: 9 in, 1 out]
    n162 = call <vilib>:"Clear Errors.vi"("error in (no error)"=w72) -> ("error out"=w71:errorcluster)  [unwired: 6 in]
  }
  n163 = while {
    tunnel: w3 -> [w365]
    tunnel: u32 500 ("milliseconds to wait") -> [w363]
    stop <- w366 stop-if-true
    # "Only read monitoring variables if the UI Main VI is connected to the RT target"
    # "Only the 'Exit' message in the UI Message Loop can stop the Monitoring Loop."
    # "Monitoring Loop"
    n164 = local read "Connected?"() -> (w364:bool)
    n165 = case shown="True" w364 {
      tunnel: w365 -> [_ w373]
      tunnel: w363 -> [w367 w368]
      frame False {
        n166 = Wait (ms)(milliseconds to wait=w367) -> ()  [unwired: 1 out]
      }
      frame True {
        # "Serialize the shared variable calls to simplify the scheduling performed by LabVIEW at runtime"
        n167 = global read "Global - UI Stream and Variable Connections.vi" "Variable References"() -> (w371:T13)
        n168 = call "UI - Read Stream from RT.vi"("Message Queue"=w373) -> ("error out"=w379:errorcluster, "Message Received?"=w369:bool, "dup Message Queue"=w372:refnum<queue>)  [unwired: 8 in]
        n169 = case shown="True" w369 {
          tunnel: w368 -> [w394 _]
          frame False {
            n170 = Wait (ms)(milliseconds to wait=w394) -> ()  [unwired: 1 out]
          }
          frame True {
            # "If a message was received, immediately read again"
          }
        }
        n171 = Unbundle By Name(w371) -> ("CPU Usage"=w386:refnum<k21>, "Contiguous Memory"=w385:refnum<k21>, "Input Values"=w384:refnum<k21>, "Output Values"=w383:refnum<k21>, "FPGA Mode"=w382:refnum<k21>, "Actual Loop Period"=w381:refnum<k21>)
        n172 = shared-variable-read(w386, w379) -> (w378:errorcluster, →"CPU Usage (%)":dbl)  [unwired: 2 out]
        n173 = shared-variable-read(w385, w378) -> (w377:errorcluster, →"Largest Contiguous Memory (bytes)":dbl)  [unwired: 2 out]
        n174 = shared-variable-read(w384, w377) -> (w376:errorcluster, w389:T12)  [unwired: 2 out]
        n175 = shared-variable-read(w383, w376) -> (w375:errorcluster, w388:T12)  [unwired: 2 out]
        n176 = shared-variable-read(w382, w375) -> (w374:errorcluster, →"Current FPGA Control Mode":T11)  [unwired: 2 out]
        n177 = shared-variable-read(w381, w374) -> (w380:errorcluster, →"Actual Loop Period (ticks)":u32)  [unwired: 2 out]
        n178 = To Double Precision Float(number=w389) -> (double precision float=→"Input Values":T4)
        n179 = To Double Precision Float(number=w388) -> (double precision float=→"Output Values":T4)
        n180 = call "UI Error Handler - Monitoring.vi"("error in (no error)"=w380, "Message Queue"=w372) -> ()  [unwired: 9 in, 1 out]
      }
    }
    n181 = global read "Global - All UI Loop Stop.vi" "All UI Loop Stop"() -> (w366:bool)
  }
  n182 = Unregister For Events(event registration refnum=w6, error in=w14) -> (error out=w7:errorcluster)
  n183 = Merge Errors(w7, w15) -> (w13:errorcluster)
  n184 = call "Destroy User Event - Stop.vi"("error in (no error)"=w13, "User Event - Stop"=w11) -> ("error out"=w4:errorcluster)  [unwired: 9 in]
  n185 = call <vilib>:"Simple Error Handler.vi"("error in (no error)"=w4) -> ()  [unwired: 4 in, 5 out]
